vi "WLAN_Example.vi"() -> ()   [LabVIEW 2016]
uses:
  Source/SA/RFmxInstr/Typedefs/Instrument Configuration.ctl
  Source/Common/Local Oscillator Sharing Mode.ctl
  Source/Common/SA Common Configuration.ctl
  Source/SA/RFmxWLAN/Typedefs/WLAN Standard Configuration.ctl
  Source/SA/RFmxWLAN/Typedefs/WLAN OFDM ModAcc Configuration.ctl
  Source/SA/RFmxWLAN/Typedefs/WLAN OFDM ModAcc Results.ctl
  Source/Common/SA Auto Level Configuration.ctl
  Source/SA/RFmxInstr/RFmxInstr.lvlib
  Source/SA/RFmxWLAN/RFmxWLAN.lvlib
  Source/Common/Common.lvlib
panel:
  out "OFDM ModAcc Results":T1 {"Composite Pilot RMS EVM Mean (dB)" format="%.2f"; "Composite Data RMS EVM Mean (dB)" format="%.2f"; "Composite RMS EVM Mean (dB)" format="%.2f"}
  out "error out":errorcluster
  in  "Tab Control":enum32{"Common", "Standard", "ModAcc"}(tab)
  in  "Resource Name":refnum<k15>="VST"
  in  "Common Configuration":T2={"Center Frequency (Hz)"=3500000000.0, "Reference Level (dBm)"=0.0, "External Attenuation (dB)"=0.0, "Trigger Enabled"=TRUE, "Digital Trigger Source"="PXI_Trig0", "Trigger Delay (s)"=0.0, "Selected Ports"=""} {"Trigger Delay (s)" format="%.2p"; "External Attenuation (dB)" format="%.2f"; "Reference Level (dBm)" format="%.2f"; "Center Frequency (Hz)" format="%.6p"}
  in  "Instrument Configuration":T3={"LO Sharing Mode"=enum."Automatic", "Frequency Reference Source"="PXI_Clk"}
  in  "Auto Level Configuration":T5={"Enabled"=TRUE, "Measurement Interval (s)"=0.01} {"Measurement Interval (s)" min=1e-06 max=100.0 format="%.2p"}
  in  "WLAN Standard Configuration":T6={"Standard"=6, "Channel Bandwidth (Hz)"=80000000.0} {"Channel Bandwidth (Hz)" items=["5M"=5000000.0, "10M"=10000000.0, "20M"=20000000.0, "40M"=40000000.0, "80M"=80000000.0, "160M"=160000000.0]; "Standard" items=["802.11a/g", "802.11b", "802.11j", "802.11p", "802.11n", "802.11ac", "802.11ax"]}
  in  "OFDM ModAcc Configuration":T7={"Acquisition Length (s)"=0.0, "Averaging Enabled"=0, "Averaging Count"=10, "Optimize Dynamic Range for EVM Enabled"=1, "Optimize Dynamic Range for EVM Margin (dB)"=0.0, "Measurement Offset (sym)"=0, "Maximum Measurement Length (sym)"=16} {"Optimize Dynamic Range for EVM Margin (dB)" format="%.2f"; "Optimize Dynamic Range for EVM Enabled" items=["False", "True"]; "Averaging Enabled" items=["False", "True"]; "Acquisition Length (s)" format="%.3p"}
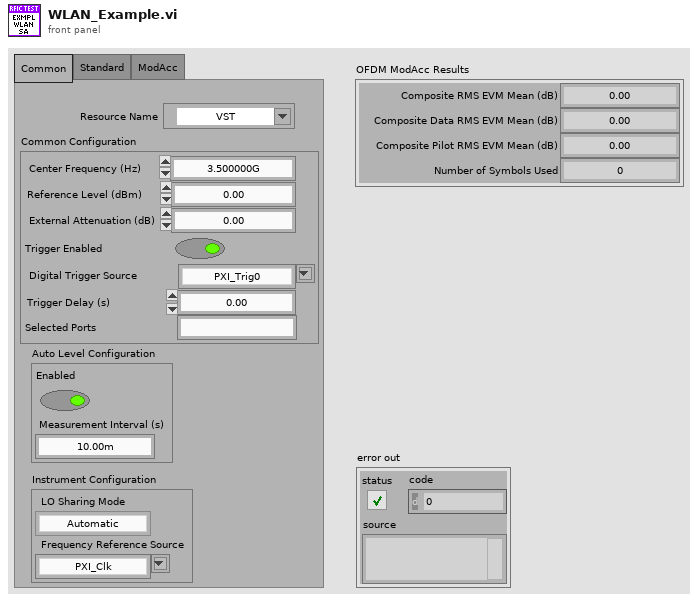
[diagram p1: front panel]
types:
  T1 = typedef "RFmxWLAN.lvlib/WLAN OFDM ModAcc Results.ctl" = cluster{"Composite RMS EVM Mean (dB)":dbl, "Composite Data RMS EVM Mean (dB)":dbl, "Composite Pilot RMS EVM Mean (dB)":dbl, "Number of Symbols Used":i32}
  T2 = typedef "Common.lvlib/SA Common Configuration.ctl" = cluster{"Center Frequency (Hz)":dbl, "Reference Level (dBm)":dbl, "External Attenuation (dB)":dbl, "Trigger Enabled":bool, "Digital Trigger Source":string, "Trigger Delay (s)":dbl, "Selected Ports":string}
  T3 = typedef "RFmxInstr.lvlib/Instrument Configuration.ctl" = cluster{"LO Sharing Mode":T4, "Frequency Reference Source":string}
  T4 = typedef "Common.lvlib/Local Oscillator Sharing Mode.ctl" = enum16{"Automatic", "None"}
  T5 = typedef "Common.lvlib/SA Auto Level Configuration.ctl" = cluster{"Enabled":bool, "Measurement Interval (s)":dbl}
  T6 = typedef "RFmxWLAN.lvlib/WLAN Standard Configuration.ctl" = cluster{"Standard":i32, "Channel Bandwidth (Hz)":dbl}
  T7 = typedef "RFmxWLAN.lvlib/WLAN OFDM ModAcc Configuration.ctl" = cluster{"Acquisition Length (s)":dbl, "Averaging Enabled":i32, "Averaging Count":i32, "Optimize Dynamic Range for EVM Enabled":i32, "Optimize Dynamic Range for EVM Margin (dB)":dbl, "Measurement Offset (sym)":i32, "Maximum Measurement Length (sym)":i32}
  T8 = enum16{"TXP", "PowerRamp", "DSSSModAcc", "OFDMModAcc", "SEM"}[]
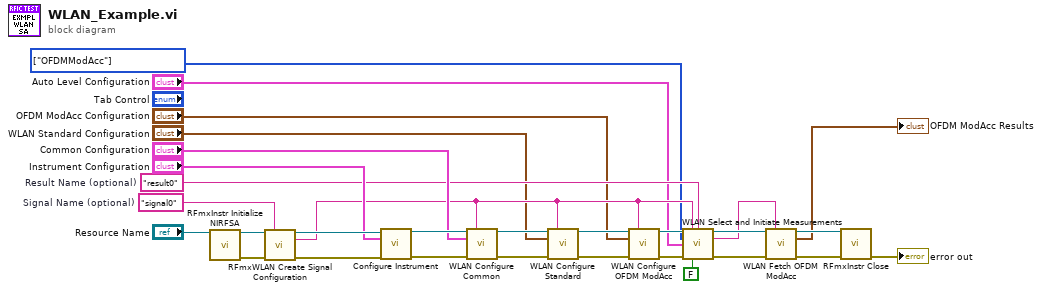
[diagram p0: block diagram]
diagram:
  w3 = T8 [enum."OFDMModAcc"] items=["TXP", "PowerRamp", "DSSSModAcc", "OFDMModAcc", "SEM"] ("Measurements")
  w14 = "result0"  # Result Name (optional)
  w22 = "signal0"  # Signal Name (optional)
  n1 = call <vilib>:"RFmxInstr Initialize NIRFSA.vi"("Resource Name"="Resource Name") -> ("Instrument Handle Out"=w23:refnum<k21>, "error out"=w28:errorcluster)  [unwired: 12 in, 1 out]
  n2 = call <vilib>:"RFmxWLAN Create Signal Configuration.vi"("Instrument Handle In"=w23, "Signal Name"=w22, "error in (no error)"=w28) -> ("Instrument Handle Out"=w21:refnum<k21>, "Selector String Out"=w15:string, "error out"=w7:errorcluster)  [unwired: 10 in]
  n3 = call "Configure Instrument.vi"("Instrument Handle In"=w21, "Instrument Configuration"="Instrument Configuration", "error in (no error)"=w7) -> ("Instrument Handle Out"=w20:refnum<k21>, "error out"=w6:errorcluster)  [unwired: 11 in]
  n4 = call "WLAN Configure Common.vi"("Instrument Handle In"=w20, "Selector String"=w15, "Common Configuration"="Common Configuration", "error in (no error)"=w6) -> ("Instrument Handle Out"=w30:refnum<k21>, "error out"=w29:errorcluster)  [unwired: 10 in]
  n5 = call "WLAN Configure Standard.vi"("Instrument Handle In"=w30, "Selector String"=w15, "WLAN Standard Configuration"="WLAN Standard Configuration", "error in (no error)"=w29) -> ("Instrument Handle Out"=w26:refnum<k21>, "error out"=w25:errorcluster)  [unwired: 10 in]
  n6 = call "WLAN Configure OFDM ModAcc.vi"("Instrument Handle In"=w26, "Selector String"=w15, "OFDM ModAcc Configuration"="OFDM ModAcc Configuration", "error in (no error)"=w25) -> ("Instrument Handle Out"=w11:refnum<k21>, "error out"=w8:errorcluster)  [unwired: 10 in]
  n7 = call "WLAN Select and Initiate Measurements.vi"("Instrument Handle In"=w11, "Selector String"=w15, "Result Name"=w14, "Measurements"=w3, "Auto Level Configuration"="Auto Level Configuration", "error in (no error)"=w8, "Enable All Traces (F)"=FALSE) -> ("Instrument Handle Out"=w17:refnum<k21>, "Selector String Out"=w13:string, "error out"=w16:errorcluster)  [unwired: 6 in]
  n8 = call "WLAN Fetch OFDM ModAcc.vi"("Instrument Handle In"=w17, "Selector String"=w13, "error in (no error)"=w16) -> ("Instrument Handle Out"=w10:refnum<k21>, "OFDM ModAcc Results"=→"OFDM ModAcc Results":T1, "error out"=w9:errorcluster)  [unwired: 10 in]
  n9 = call <vilib>:"RFmxInstr Close.vi"("Instrument Handle In"=w10, "error in (no error)"=w9) -> ("error out"=→"error out":errorcluster)  [unwired: 13 in]
